vi "FIO.vi"(0 "System no.":i32=1 min=1 step=1, 1 "Board":i32=1 min=1 max=5 step=1, 2 "Axis 1 to scan":string, 3 "Axis 2 to scan":string, 4 "Max. area \nsize, mm":dbl=0.2 format="%.4f", 5 "error in":errorcluster, 6 "Treshold level":dbl=0.1 format="%.3f", 7 "Step size\nlinear spiral":dbl=0.01 format="%.4f", 8 "Max. area \nsize 2, mm":dbl=0.2 format="%.4f", 9 "Angular area, \ndeg":dbl=0.2 format="%.4f", 10 "Use #7 polling?":bool, 11 "Timeout (s)":dbl=300.0 min=1.0 max=4.0 step=1.0 format="%.2f", 12 "Stop refnum":refnum<vi>) -> (14 "Scan successful?":bool, 19 "error out":errorcluster)   [LabVIEW 2020]
doc: "Performs a fast input/output automated alignment procedure in specified axes, waits until scan is ready (using #7 polling if checked) and indicates whether scan was successful or not. If Refnum stop or Local stop is TRUE, VI sends #24 and stops. \n\"Timeout\" is only valid if \"Use #7 polling\" is FALSE. \n\nC-887, F-206, M-8X0: : For GCS syntax version = GCS 2.0 or higher (check with CSV?.vi. If CSV?.vi is not supported, syntax version is GCS 1.0), VI calls FSS? automatically to determine if scan was successful or not. Use #7 polling = FALSE. Max. area size 2 must be identical to Max. area size."
uses:
  Communication.llb/Syntax.ctl
  Communication.llb/Global1.vi
panel:
  in  "Local stop":bool
  # "Performs a fast input/output automated alignment procedure in\nspecified axes, waits until scan is ready (using #7 polling if checked) \nand indicates whether scan was successful or not.  If Stop refnum or \nLocal stop is TRUE, VI sends #24 and stops. \"Timeout\"  is only valid if \n\"Use #7 polling\" is FALSE."
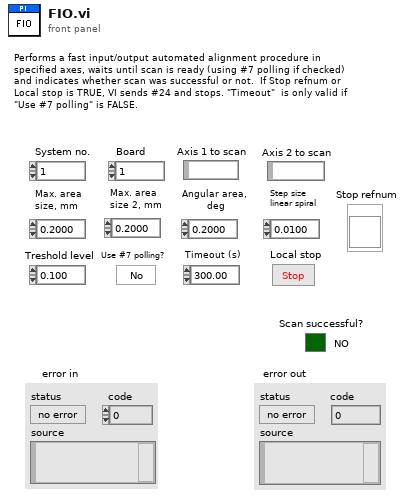
[diagram p1: front panel]
types:
  T1 = typedef "Syntax.ctl" = enum16{"GCS 1.0", "GCS 2.0", "GCS 3.0"}
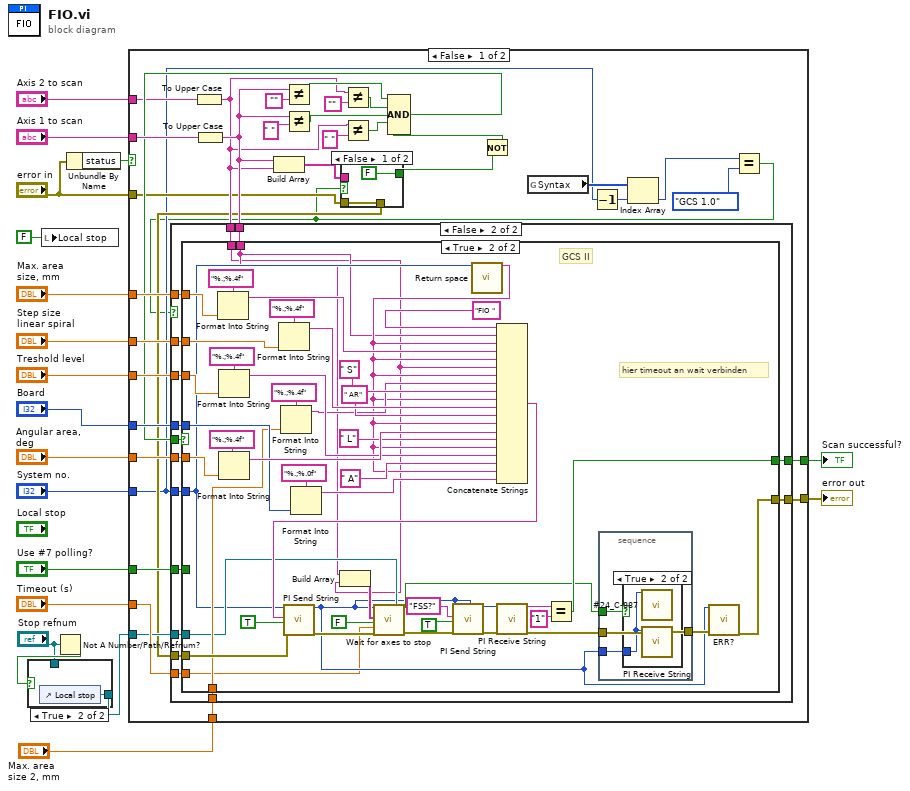
[diagram p0: block diagram]
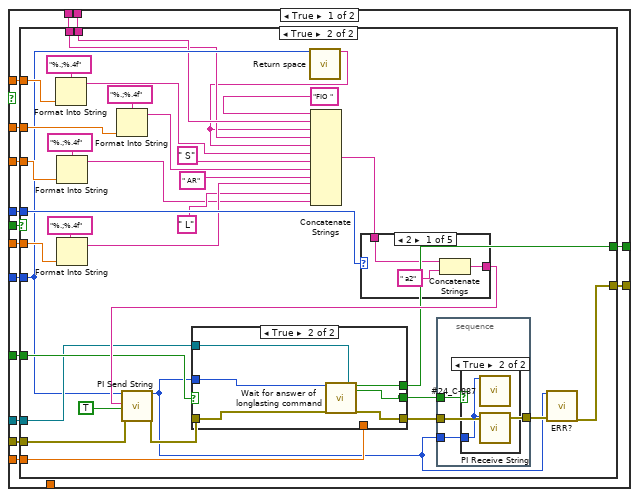
[diagram p3: hidden frame]
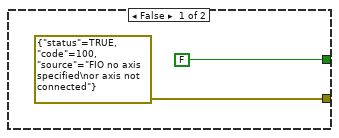
[diagram p4: hidden frame]
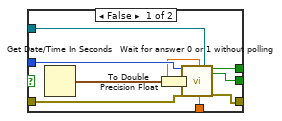
[diagram p6: hidden frame]
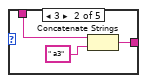
[diagram p7: hidden frame]
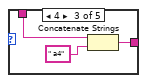
[diagram p8: hidden frame]
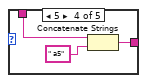
[diagram p9: hidden frame]
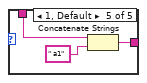
[diagram p10: hidden frame]
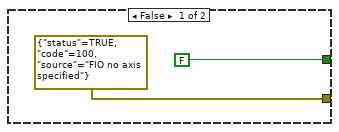
[diagram p11: hidden frame]
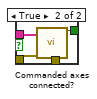
[diagram p13: hidden frame]
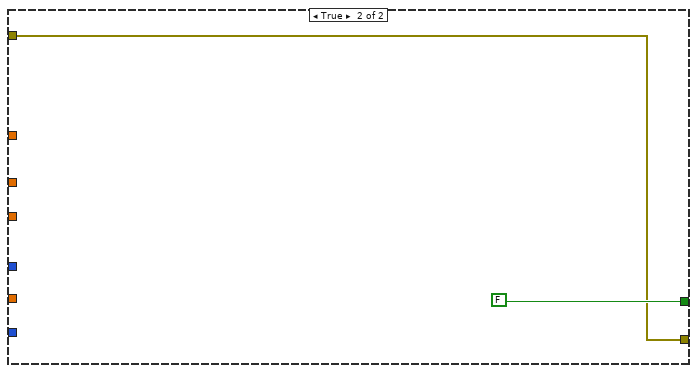
[diagram p14: hidden frame]
diagram:
  n1 = local write "Local stop"(FALSE ("Local stop")) -> ()
  n2 = Not A Number/Path/Refnum?(number/path/refnum="Stop refnum") -> (NaN/Path/Refnum?=w4:bool)
  n3 = case shown="True" w4 {
    tunnel: [w20 w21] -> w2
    tunnel: "Stop refnum" -> [w20 _]
    frame False {
    }
    frame True {
      n4 = control-ref of="Local stop"() -> (w21:refnum<vi>)
    }
  }
  n5 = Unbundle By Name("error in") -> ("status"=w14:bool)
  n6 = case shown="False" w14 {
    tunnel: "System no." -> [w26 _]
    tunnel: [w47 w216] -> w18
    tunnel: "Axis 1 to scan" -> [w56 _]
    tunnel: [w46 FALSE] -> w16
    tunnel: "error in" -> [w27 w216]
    tunnel: "Board" -> [w52 _]
    tunnel: "Max. area \nsize, mm" -> [w51 _]
    tunnel: "Step size\nlinear spiral" -> [w50 _]
    tunnel: "Treshold level" -> [w49 _]
    tunnel: "Axis 2 to scan" -> [w43 _]
    tunnel: "Use #7 polling?" -> [w36 _]
    tunnel: "Timeout (s)" -> [w35 _]
    tunnel: "Angular area, \ndeg" -> [w34 _]
    tunnel: w2 -> [w33 _]
    tunnel: "Max. area \nsize 2, mm" -> [w23 _]
    frame False {
      n7 = To Upper Case(1:w43) -> (0:w37:string)
      n8 = To Upper Case(1:w56) -> (0:w38:string)
      n9 = Build Array(w38, w37) -> (w24:string[])
      n10 = Not Equal?(x=w38, y="") -> (x != y?=w53:bool)
      n11 = Not Equal?(x=w38, y=" ") -> (x != y?=w41:bool)
      n12 = Not Equal?(x=w37, y="") -> (x != y?=w40:bool)
      n13 = Not Equal?(x=w37, y=" ") -> (x != y?=w39:bool)
      n14 = global read "Global1.vi" "Syntax"() -> (w30:T1[])
      n15 = Decrement(x=w26) -> (x-1=w31:i32)
      n16 = Index Array(array=w30, index=w31) -> (element=w32:T1)
      n17 = Equal?(x=w32, y=Syntax."GCS 1.0") -> (x = y?=w25:bool)
      n18 = case shown="False" w25 {
        tunnel: w27 -> [w211 w215]
        tunnel: [w211 w214] -> w28
        tunnel: [FALSE ("Controller error") w213] -> w29
        tunnel: w24 -> [_ w212]
        frame False {
        }
        frame True {
          n19 = call "Commanded axes connected?.vi"("Commanded axes"=w212, "error in"=w215) -> ("Controller error"=w213:bool, "error out"=w214:errorcluster)  [unwired: 1 in, 15 out]
        }
      }
      n20 = Not(x=w29) -> (.not. x?=w45:bool)
      n21 = Compound Arithmetic op=AND(w53, w40, w41, w39, w45) -> (w48:bool)
      n22 = case shown="False" w25 {
        tunnel: w52 -> [w71 w157]
        tunnel: w51 -> [w70 w156]
        tunnel: w50 -> [w69 w155]
        tunnel: w49 -> [w68 w154]
        tunnel: w48 -> [w67 w153]
        tunnel: w26 -> [w66 w152]
        tunnel: [w65 w151] -> w47
        tunnel: [w64 w150] -> w46
        tunnel: w38 -> [w63 w149]
        tunnel: w37 -> [w62 w148]
        tunnel: w36 -> [w61 w147]
        tunnel: w35 -> [w60 w146]
        tunnel: w34 -> [w59 w145]
        tunnel: w33 -> [w58 w144]
        tunnel: w28 -> [w57 w143]
        tunnel: w23 -> [_ w142]
        frame True {
          n23 = case shown="True" w67 {
            tunnel: w71 -> [_ w107]
            tunnel: w70 -> [_ w92]
            tunnel: w69 -> [_ w96]
            tunnel: w63 -> [_ w76]
            tunnel: w68 -> [_ w98]
            tunnel: w57 -> [_ w104]
            tunnel: w66 -> [_ w78]
            tunnel: [errorcluster {"status"=TRUE, "code"=100, "source"="FIO no axis specified\nor axis not connected"} ("error out") w88] -> w65
            tunnel: [FALSE w101] -> w64
            tunnel: w62 -> [_ w75]
            tunnel: w61 -> [_ w94]
            tunnel: w60 -> [_ w93]
            tunnel: w59 -> [_ w91]
            tunnel: w58 -> [_ w80]
            frame False {
            }
            frame True {
              n24 = Format Into String(format string="%.;%.4f" ("Format String"), w92) -> (resulting string=w95:string)  [unwired: 2 in, 1 out]
              n25 = Format Into String(format string="%.;%.4f" ("Format String"), w98) -> (resulting string=w81:string)  [unwired: 2 in, 1 out]
              n26 = Format Into String(format string="%.;%.4f" ("Format String"), w91) -> (resulting string=w83:string)  [unwired: 2 in, 1 out]
              n27 = Format Into String(format string="%.;%.4f" ("Format String"), w96) -> (resulting string=w85:string)  [unwired: 2 in, 1 out]
              n28 = call "Return space.vi"("System no."=w78) -> ("String out"=w74:string)  [unwired: 1 in, 17 out]
              n29 = Concatenate Strings("FIO ", w76, w74, w75, w74, w95, " S", w85, " AR", w83, " L", w81) -> (w106:string)
              n30 = case shown="2" w107 {
                tunnel: w106 -> [w129 w132 w135 w138 w141]
                tunnel: [w127 w130 w133 w136 w139] -> w105
                frame 2 {
                  n31 = Concatenate Strings(w129, " a2" ("Substring")) -> (w127:string)
                }
                frame 3 {
                  n32 = Concatenate Strings(w132, " a3" ("Substring")) -> (w130:string)
                }
                frame 4 {
                  n33 = Concatenate Strings(w135, " a4" ("Substring")) -> (w133:string)
                }
                frame 5 {
                  n34 = Concatenate Strings(w138, " a5" ("Substring")) -> (w136:string)
                }
                frame 1, Default {
                  n35 = Concatenate Strings(w141, " a1" ("Substring")) -> (w139:string)
                }
              }
              n36 = call "PI Send String.vi"("System no."=w78, "String to send"=w105, "Attach termination char.?"=TRUE ("Attach Linefeed?"), "error in"=w104) -> ("error out"=w102:errorcluster)  [unwired: 15 out]
              n37 = case shown="True" w94 {
                tunnel: w78 -> [w120 w126]
                tunnel: w102 -> [w119 w125]
                tunnel: [w118 w124] -> w90
                tunnel: [w117 w123] -> w101
                tunnel: w93 -> [w115 _]
                tunnel: w80 -> [w114 w122]
                tunnel: [w113 w121] -> w79
                frame False {
                  n38 = Get Date/Time In Seconds() -> (seconds since 1Jan1904=w112:timestamp)
                  n39 = To Double Precision Float(number=w112) -> (double precision float=w116:dbl)
                  n40 = call "Wait for answer 0 or 1 without polling.vi"("System no."=w120, "error in"=w119, "Start time"=w116, "Timeout (s)"=w115, "Stop refnum"=w114) -> ("Scan successful?"=w117:bool, "Stopped"=w113:bool, "error out"=w118:errorcluster)  [unwired: 12 out]
                }
                frame True {
                  n41 = call "Wait for answer of longlasting command.vi"("System no."=w126, "error in"=w125, "Stop refnum"=w122) -> ("Answer"=w123:bool, "Stopped"=w121:bool, "error out"=w124:errorcluster)  [unwired: 14 out]
                }
              }
              n42 = stacked-sequence {
                tunnel: w78 -> [w110]
                tunnel: w90 -> [w109]
                tunnel: [w109] -> w89
                tunnel: w79 -> [w108]
                frame #0 {
                  n43 = case shown="True" w108 {
                    tunnel: w110 -> [_ w111]
                    frame False {
                    }
                    frame True {
                      n44 = call "#24_C-887.vi"("System no."=w111) -> ()  [unwired: 1 in, 18 out]
                      n45 = call "PI Receive String.vi"("System no."=w111) -> ()  [unwired: 2 in, 17 out]
                    }
                  }
                }
              }
              n46 = call "ERR?.vi"("System no."=w78, "error in"=w89) -> ("error out"=w88:errorcluster)  [unwired: 17 out]
            }
          }
        }
        frame False {
          n47 = case shown="True" w153 {
            tunnel: w157 -> [_ w185]
            tunnel: w156 -> [_ w198]
            tunnel: w155 -> [_ w199]
            tunnel: w149 -> [_ w162]
            tunnel: w154 -> [_ w201]
            tunnel: w143 -> [_ w205]
            tunnel: w152 -> [_ w163]
            tunnel: [errorcluster {"status"=TRUE, "code"=100, "source"="FIO no axis specified"} ("error out") w195] -> w151
            tunnel: [FALSE w166] -> w150
            tunnel: w148 -> [_ w161]
            tunnel: w147 -> [_ _]
            tunnel: w146 -> [_ w160]
            tunnel: w145 -> [_ w197]
            tunnel: w144 -> [_ w164]
            tunnel: w142 -> [_ w180]
            frame False {
            }
            frame True {
              # "hier timeout an wait verbinden"
              # "GCS II"
              n48 = Format Into String(format string="%.;%.4f" ("Format String"), w198) -> (resulting string=w179:string)  [unwired: 2 in, 1 out]
              n49 = Format Into String(format string="%.;%.4f" ("Format String"), w201) -> (resulting string=w188:string)  [unwired: 2 in, 1 out]
              n50 = Format Into String(format string="%.;%.4f" ("Format String"), w197) -> (resulting string=w190:string)  [unwired: 2 in, 1 out]
              n51 = Format Into String(format string="%.;%.4f" ("Format String"), w199) -> (resulting string=w192:string)  [unwired: 2 in, 1 out]
              n52 = Format Into String(format string="%.;%.4f" ("Format String"), w180) -> (resulting string=w178:string)  [unwired: 2 in, 1 out]
              n53 = Format Into String(format string="%.;%.0f" ("Format String"), w185) -> (resulting string=w184:string)  [unwired: 2 in, 1 out]
              n54 = Build Array(w162, w161) -> (w175:string[])
              n55 = call "Return space.vi"("System no."=w163) -> ("String out"=w177:string)  [unwired: 1 in, 17 out]
              n56 = Concatenate Strings("FIO ", w162, w177, w179, w177, w161, w177, w178, " S", w177, w192, " AR", w177, w190, " L", w177, w188, " A", w177, w184) -> (w182:string)
              n57 = call "PI Send String.vi"("System no."=w163, "String to send"=w182, "Attach termination char.?"=TRUE ("Attach Linefeed?"), "error in"=w205) -> ("error out"=w168:errorcluster)  [unwired: 15 out]
              n58 = call "Wait for axes to stop.vi"("System no."=w163, "Axes to wait for"=w175, "With status bit polling?"=FALSE, "Timeout (s)"=w160, "error in"=w168, "Stop refnum"=w164) -> ("Stopped"=w165:bool, "error out"=w172:errorcluster)  [unwired: 1 in, 11 out]
              n59 = call "PI Send String.vi"("System no."=w163, "String to send"="FSS?", "Attach termination char.?"=TRUE ("Attach Linefeed?"), "error in"=w172) -> ("error out"=w171:errorcluster)  [unwired: 15 out]
              n60 = call "PI Receive String.vi"("System no."=w163, "error in"=w171) -> ("String read"=w169:string, "error out"=w167:errorcluster)  [unwired: 1 in, 15 out]
              n61 = Equal?(x=w169, y="1") -> (x = y?=w166:bool)
              n62 = stacked-sequence {
                tunnel: w163 -> [w208]
                tunnel: w167 -> [w207]
                tunnel: [w207] -> w196
                tunnel: w165 -> [w206]
                frame #0 {
                  n63 = case shown="True" w206 {
                    tunnel: w208 -> [_ w209]
                    frame False {
                    }
                    frame True {
                      n64 = call "#24_C-887.vi"("System no."=w209) -> ()  [unwired: 1 in, 18 out]
                      n65 = call "PI Receive String.vi"("System no."=w209) -> ()  [unwired: 2 in, 17 out]
                    }
                  }
                }
              }
              n66 = call "ERR?.vi"("System no."=w163, "error in"=w196) -> ("error out"=w195:errorcluster)  [unwired: 17 out]
            }
          }
        }
      }
    }
    frame True {
    }
  }
  "error out" <- w18
  "Scan successful?" <- w16
